vi "vision-board converter to room.vi"(1 "Array in":string[][](array[string])) -> (0 "Array out":string[][](array[string]))   [LabVIEW 2019]
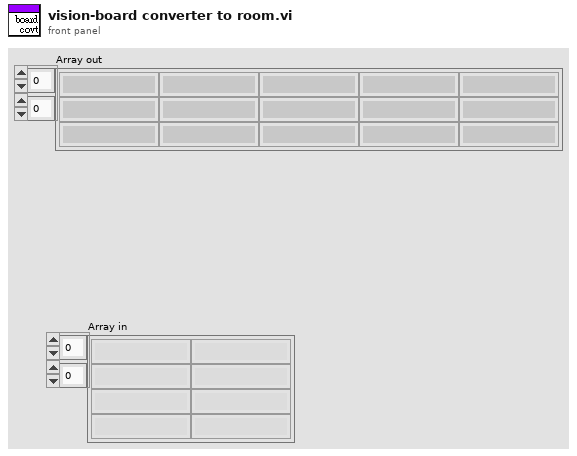
[diagram p1: front panel]
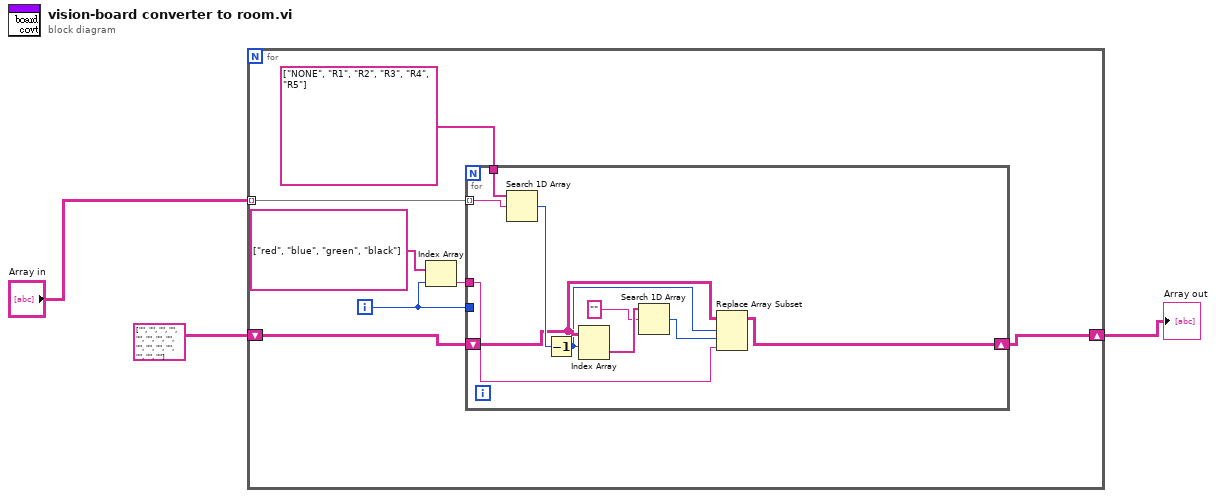
[diagram p0: block diagram]
diagram:
  n1 = for {
    tunnel: "Array in" -> [w10] mode=indexing
    shift-right: [w4] -> w1
    shift-left: string[][] [["", "", ""], ["", "", ""], ["", "", ""], ["", "", ""], ["", "", ""]] -> [w5]
    i -> [w6]
    n2 = Index Array(array=string[] ["red", "blue", "green", "black"], index=w6) -> (element=w7:string)
    n3 = for {
      tunnel: w10 -> [w19] mode=indexing
      tunnel: string[] ["NONE", "R1", "R2", "R3", "R4", "R5"] -> [w20]
      tunnel: w7 -> [w12]
      tunnel: w6 -> [_]
      shift-right: [w11] -> w4
      shift-left: w5 -> [w15]
      n4 = Search 1D Array(1D array=w20, element=w19) -> (index of element=w18:i32)  [unwired: 1 in]
      n5 = Decrement(x=w18) -> (x-1=w14:i32)
      n6 = Index Array(array=w15, index (row)=w14) -> (element=w17:string[])  [unwired: 1 in]
      n7 = Search 1D Array(1D array=w17, element="") -> (index of element=w13:i32)  [unwired: 1 in]
      n8 = Replace Array Subset(array=w15, new element=w12, index (row)=w14, index (col)=w13) -> (w11:string[][])
    }
  }
  "Array out" <- w1
